vi "ArduinoNano33IOTCompile.vi"(8 "ino file":path, 9 "Packages":path, 10 "bin location to upload":path, 11 "Java":path) -> (0 "standard error":string, 3 "standard output":string)   [LabVIEW 2019]
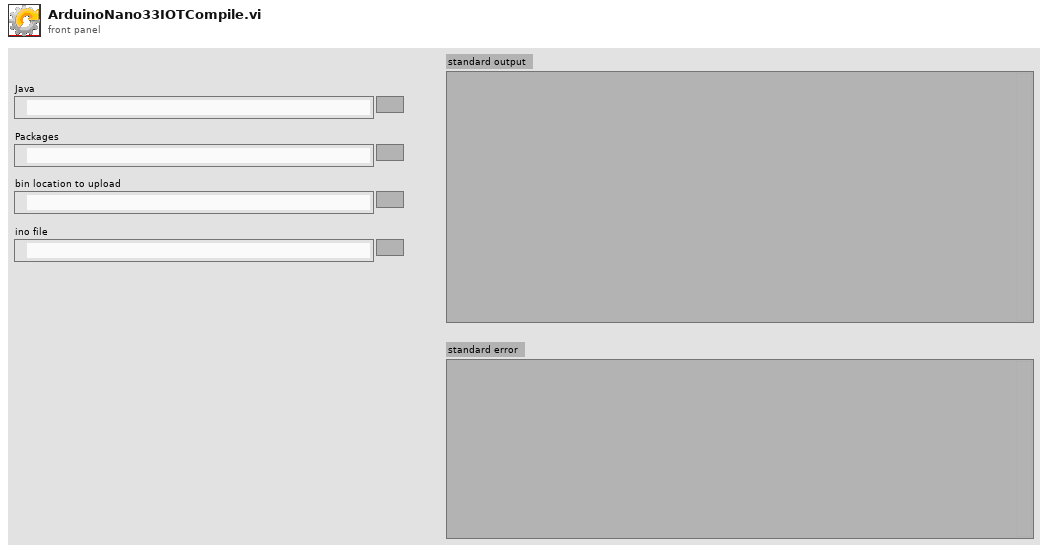
[diagram p1: front panel]
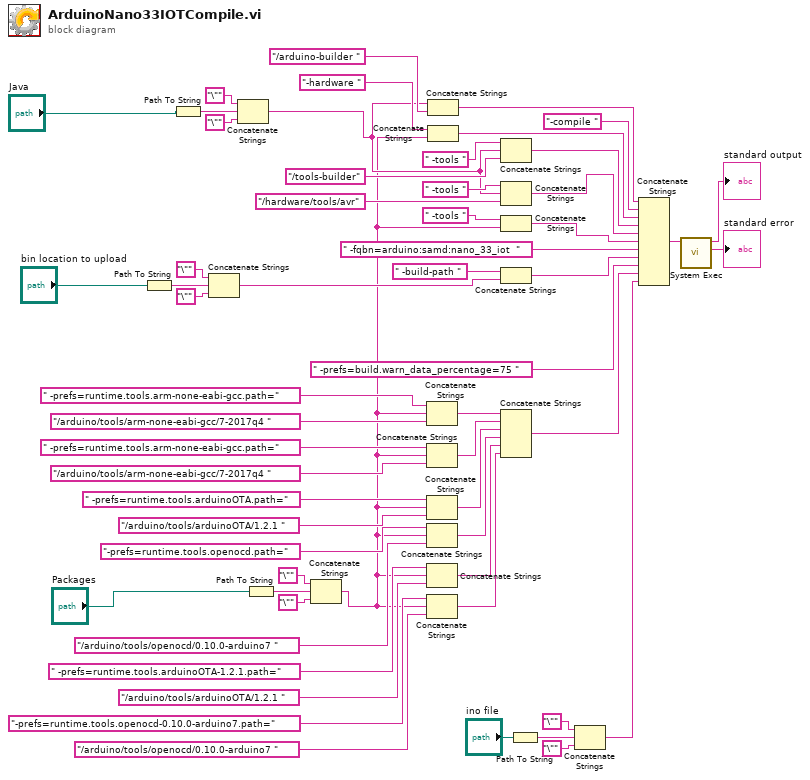
[diagram p0: block diagram]
diagram:
  n1 = Path To String(path="bin location to upload") -> (string=w16:string)
  n2 = Path To String(path="Java") -> (string=w8:string)
  n3 = Concatenate Strings("\"" ("string"), w16, "\"" ("string")) -> (w15:string)
  n4 = Concatenate Strings("\"" ("string"), w8, "\"" ("string")) -> (w6:string)
  n5 = Path To String(path="Packages") -> (string=w3:string)
  n6 = Concatenate Strings("\"" ("string"), w3, "\"" ("string")) -> (w1:string)
  n7 = Concatenate Strings(" -prefs=runtime.tools.arm-none-eabi-gcc.path=" ("string"), w1, "/arduino/tools/arm-none-eabi-gcc/7-2017q4 " ("string")) -> (w24:string)
  n8 = Concatenate Strings(" -prefs=runtime.tools.arm-none-eabi-gcc.path=" ("string"), w1, "/arduino/tools/arm-none-eabi-gcc/7-2017q4 " ("string")) -> (w29:string)
  n9 = Concatenate Strings(" -prefs=runtime.tools.arduinoOTA.path=" ("string"), w1, "/arduino/tools/arduinoOTA/1.2.1 " ("string")) -> (w28:string)
  n10 = Concatenate Strings("-prefs=runtime.tools.openocd.path=" ("string"), w1, "/arduino/tools/openocd/0.10.0-arduino7 " ("string")) -> (w27:string)
  n11 = Concatenate Strings(" -prefs=runtime.tools.arduinoOTA-1.2.1.path=" ("string"), w1, "/arduino/tools/arduinoOTA/1.2.1 " ("string")) -> (w26:string)
  n12 = Concatenate Strings("-prefs=runtime.tools.openocd-0.10.0-arduino7.path=" ("string"), w1, "/arduino/tools/openocd/0.10.0-arduino7 " ("string")) -> (w25:string)
  n13 = Concatenate Strings(w6, "/arduino-builder " ("string")) -> (w54:string)
  n14 = Concatenate Strings("-hardware " ("string"), w1) -> (w39:string)
  n15 = Concatenate Strings(" -tools " ("string"), w6, "/tools-builder" ("string")) -> (w38:string)
  n16 = Concatenate Strings(" -tools " ("string"), w6, "/hardware/tools/avr" ("string")) -> (w11:string)
  n17 = Concatenate Strings(" -tools " ("string"), w1) -> (w12:string)
  n18 = Concatenate Strings(" -build-path " ("string"), w15) -> (w36:string)
  n19 = Concatenate Strings(w24, w29, w28, w27, w26, w25) -> (w23:string)
  n20 = Path To String(path="ino file") -> (string=w13:string)
  n21 = Concatenate Strings("\"" ("string"), w13, "\"" ("string")) -> (w14:string)
  n22 = Concatenate Strings(w54, "-compile " ("string"), w39, w38, w11, w12, " -fqbn=arduino:samd:nano_33_iot  " ("string"), w36, " -prefs=build.warn_data_percentage=75 " ("string"), w23, w14) -> (w58:string)
  n23 = call <vilib>:"System Exec.vi"("command line"=w58) -> ("standard error"=→"standard error":string, "standard output"=→"standard output":string)  [unwired: 7 in, 2 out]
